vi "Example_OE2011 GPIB Control.vi"() -> ()   [LabVIEW 2011]
panel:
  in  "error in (no error)":errorcluster
  out "Parameter Values":T1
  in  "OE2011_Query Multi Data":T2={"Query Type 1"=0, "Query Type 5"=32, "Query Type 4"=3, "Query Type 3"=2, "Query Type 2"=1, "Query Type 6"=36} {"Query Type 6" items=["X-Demod1", "Y-Demod1", "R-Demod1", "Theta-Demod1", "X-Demod2", "Y-Demod2", "R-Demod2", "Theta-Demod2", "X-Demod3", "Y-Demod3", "R-Demod3", "Theta-Demod3", "X-Demod4", "Y-Demod4", "R-Demod4", "Theta-Demod4", "X-Demod5", "Y-Demod5", "R-Demod5", "Theta-Demod5", "X-Demod6", "Y-Demod6", "R-Demod6", "Theta-Demod6", "X-Demod7", "Y-Demod7", "R-Demod7", "Theta-Demod7", "X-Demod8", "Y-Demod8", "R-Demod8", "Theta-Demod8", "Xnoisd-Demod1", "Ynoisd-Demod1", "Xnoisd-Demod5", "Ynoisd-Demod5", "Frequency-OSC1", "Frequency-OSC2", "AUXIN1", "AUXIN2", "AUXIN3", "AUXIN4"]; "Query Type 2" items=["X-Demod1", "Y-Demod1", "R-Demod1", "Theta-Demod1", "X-Demod2", "Y-Demod2", "R-Demod2", "Theta-Demod2", "X-Demod3", "Y-Demod3", "R-Demod3", "Theta-Demod3", "X-Demod4", "Y-Demod4", "R-Demod4", "Theta-Demod4", "X-Demod5", "Y-Demod5", "R-Demod5", "Theta-Demod5", "X-Demod6", "Y-Demod6", "R-Demod6", "Theta-Demod6", "X-Demod7", "Y-Demod7", "R-Demod7", "Theta-Demod7", "X-Demod8", "Y-Demod8", "R-Demod8", "Theta-Demod8", "Xnoisd-Demod1", "Ynoisd-Demod1", "Xnoisd-Demod5", "Ynoisd-Demod5", "Frequency-OSC1", "Frequency-OSC2", "AUXIN1", "AUXIN2", "AUXIN3", "AUXIN4"]; "Query Type 3" items=["X-Demod1", "Y-Demod1", "R-Demod1", "Theta-Demod1", "X-Demod2", "Y-Demod2", "R-Demod2", "Theta-Demod2", "X-Demod3", "Y-Demod3", "R-Demod3", "Theta-Demod3", "X-Demod4", "Y-Demod4", "R-Demod4", "Theta-Demod4", "X-Demod5", "Y-Demod5", "R-Demod5", "Theta-Demod5", "X-Demod6", "Y-Demod6", "R-Demod6", "Theta-Demod6", "X-Demod7", "Y-Demod7", "R-Demod7", "Theta-Demod7", "X-Demod8", "Y-Demod8", "R-Demod8", "Theta-Demod8", "Xnoisd-Demod1", "Ynoisd-Demod1", "Xnoisd-Demod5", "Ynoisd-Demod5", "Frequency-OSC1", "Frequency-OSC2", "AUXIN1", "AUXIN2", "AUXIN3", "AUXIN4"]; "Query Type 4" items=["X-Demod1", "Y-Demod1", "R-Demod1", "Theta-Demod1", "X-Demod2", "Y-Demod2", "R-Demod2", "Theta-Demod2", "X-Demod3", "Y-Demod3", "R-Demod3", "Theta-Demod3", "X-Demod4", "Y-Demod4", "R-Demod4", "Theta-Demod4", "X-Demod5", "Y-Demod5", "R-Demod5", "Theta-Demod5", "X-Demod6", "Y-Demod6", "R-Demod6", "Theta-Demod6", "X-Demod7", "Y-Demod7", "R-Demod7", "Theta-Demod7", "X-Demod8", "Y-Demod8", "R-Demod8", "Theta-Demod8", "Xnoisd-Demod1", "Ynoisd-Demod1", "Xnoisd-Demod5", "Ynoisd-Demod5", "Frequency-OSC1", "Frequency-OSC2", "AUXIN1", "AUXIN2", "AUXIN3", "AUXIN4"]; "Query Type 5" items=["X-Demod1", "Y-Demod1", "R-Demod1", "Theta-Demod1", "X-Demod2", "Y-Demod2", "R-Demod2", "Theta-Demod2", "X-Demod3", "Y-Demod3", "R-Demod3", "Theta-Demod3", "X-Demod4", "Y-Demod4", "R-Demod4", "Theta-Demod4", "X-Demod5", "Y-Demod5", "R-Demod5", "Theta-Demod5", "X-Demod6", "Y-Demod6", "R-Demod6", "Theta-Demod6", "X-Demod7", "Y-Demod7", "R-Demod7", "Theta-Demod7", "X-Demod8", "Y-Demod8", "R-Demod8", "Theta-Demod8", "Xnoisd-Demod1", "Ynoisd-Demod1", "Xnoisd-Demod5", "Ynoisd-Demod5", "Frequency-OSC1", "Frequency-OSC2", "AUXIN1", "AUXIN2", "AUXIN3", "AUXIN4"]; "Query Type 1" items=["X-Demod1", "Y-Demod1", "R-Demod1", "Theta-Demod1", "X-Demod2", "Y-Demod2", "R-Demod2", "Theta-Demod2", "X-Demod3", "Y-Demod3", "R-Demod3", "Theta-Demod3", "X-Demod4", "Y-Demod4", "R-Demod4", "Theta-Demod4", "X-Demod5", "Y-Demod5", "R-Demod5", "Theta-Demod5", "X-Demod6", "Y-Demod6", "R-Demod6", "Theta-Demod6", "X-Demod7", "Y-Demod7", "R-Demod7", "Theta-Demod7", "X-Demod8", "Y-Demod8", "R-Demod8", "Theta-Demod8", "Xnoisd-Demod1", "Ynoisd-Demod1", "Xnoisd-Demod5", "Ynoisd-Demod5", "Frequency-OSC1", "Frequency-OSC2", "AUXIN1", "AUXIN2", "AUXIN3", "AUXIN4"]}
  in  "OE2011_Configure Input Filter":T3 {"Input Range" items=["2V", "500mV", "200mV", "50mV", "20mV", "5mV", "2mV"]; "Input Coupling" items=["AC", "DC"]; "Input Shield Grounding" items=["Float", "Ground"]; "Input Source" items=["A", "B", "Current"]}
  out "Read Buffer":string
  in  "VISA resource name":refnum<visa-resource-name>
  out "Error out":errorcluster caption="error out"
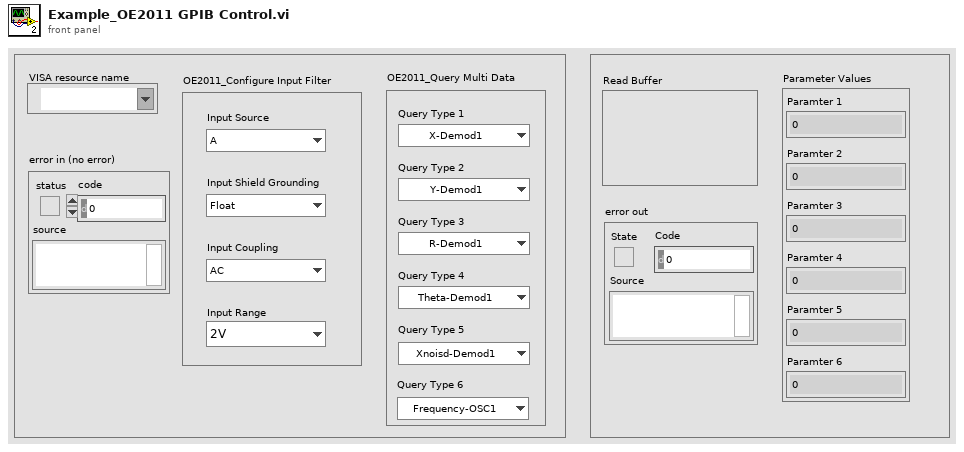
[diagram p1: front panel]
types:
  T1 = cluster{"Paramter 1":dbl, "Paramter 2":dbl, "Paramter 3":dbl, "Paramter 4":dbl, "Paramter 5":dbl, "Paramter 6":dbl}
  T2 = cluster{"Query Type 1":u16, "Query Type 5":u16, "Query Type 4":u16, "Query Type 3":u16, "Query Type 2":u16, "Query Type 6":u16}
  T3 = cluster{"Input Source":u16, "Input Shield Grounding ":u16, "Input Coupling ":u16, "Input Range":u16}
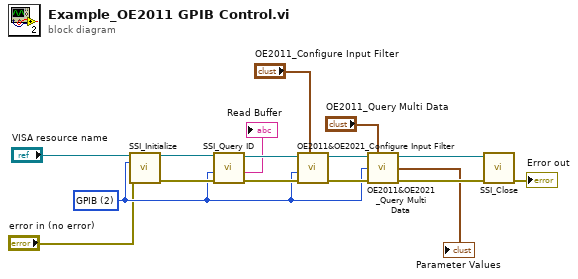
[diagram p0: block diagram]
diagram:
  w6 = u16 2 items=["USB", "RS232", "GPIB", "Ethernet"] ("Remote Mode")
  n1 = call "SSI_Initialize.vi"("VISA resource name"="VISA resource name", "Remote Mode"=w6, "error in (no error)"="error in (no error)") -> ("VISA resource name out"=w16:refnum<visa-resource-name>, "error out"=w15:errorcluster)  [unwired: 10 in, 1 out]
  n2 = call "SSI_Query ID.vi"("Error in (no error)"=w15, "Remote Mode"=w6, "VISA resource name"=w16) -> ("Error out"=w14:errorcluster, "Read Buffer"=→"Read Buffer":string, "VISA resource  out"=w13:refnum<visa-resource-name>)  [unwired: 5 in, 1 out]
  n3 = call "OE2011&OE2021_Configure Input Filter.vi"("OE2011&OE2021_\nConfigure Input Filter"="OE2011_Configure Input Filter", "Error in (no error)"=w14, "Remote Mode"=w6, "VISA resource name"=w13) -> ("Error out"=w11:errorcluster, "VISA resource  out"=w12:refnum<visa-resource-name>)  [unwired: 4 in, 2 out]
  n4 = call "OE2011&OE2021_Query Multi Data.vi"("VISA resource name"=w12, "OE2011&OE2021_\nQuery Multi Data"="OE2011_Query Multi Data", "Remote Mode"=w6, "Error in (no error)"=w11) -> ("VISA resource  out"=w9:refnum<visa-resource-name>, "Parameter Values"=→"Parameter Values":T1, "Error out"=w10:errorcluster)  [unwired: 7 in, 2 out]
  n5 = call "SSI_Close.vi"("Error in (no error)"=w10, "VISA resource name"=w9) -> ("Error out"=→"Error out":errorcluster)  [unwired: 5 in]
